vi "Test_ReadFast.vi"() -> (3 "Passed?":bool)   [LabVIEW 2017, in "WordManipulationTests.lvlib"]
uses:
  WordManipulationTests.lvlib
  SoftmotionClass/SoftmotionAxis/SoftmotionAxis.lvclass
  <vilib>/Motion/PropertyNodes/nimc.createStraightLineMoveInstance.axis.vi
  <vilib>/Motion/PropertyNodes/nimc.destroyInterfaceInstance.vi
  Utilities/WordManipulationLibrary.lvlib
  <resource>/objmgr/nimcai.rc
  Utilities/Bit Manipulation.lvlib
panel:
  out "appended array":dbl[](array[numeric])
  out "Velocity Feedback":dbl
  out "Position Feedback":dbl[](array[numeric])
  in  "Positions":dbl[](array[numeric])=[1000.0]
  in  "Velocity":dbl=1000.0
  in  "Acceleration":dbl=10000.0
  in  "Acceleration Jerk":dbl=1000.0
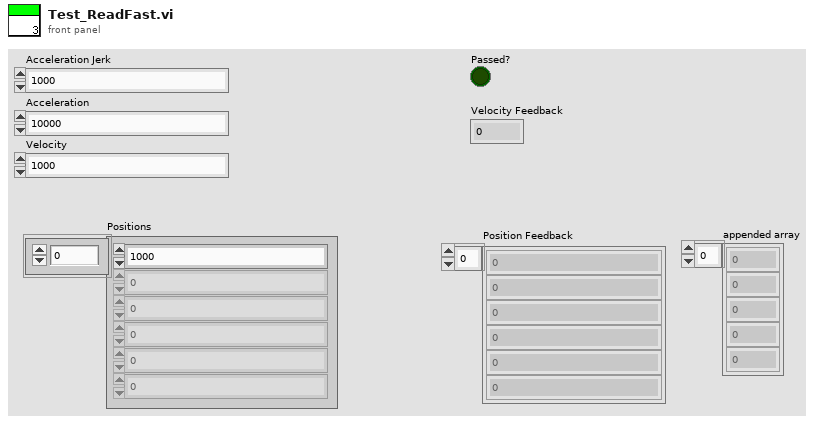
[diagram p1: front panel]
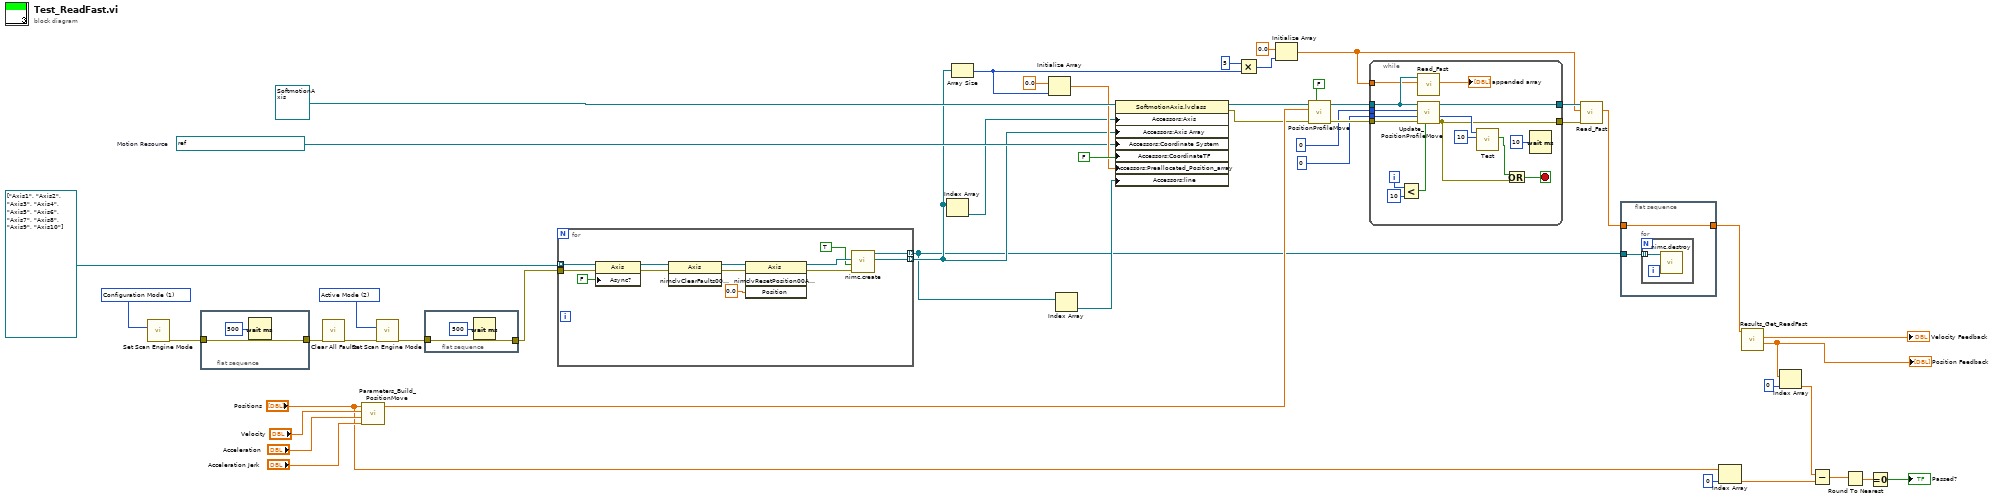
[diagram p0: block diagram]
diagram:
  w13 = 2 items=["Configuration Mode"=1, "Active Mode"=2] ("mode (Active Mode)")
  w15 = 1 items=["Configuration Mode"=1, "Active Mode"=2] ("mode (Active Mode)")
  w37 = refnum<k21> "nism://My Computer/Cord1"  # Motion Resource
  n1 = call <vilib>:"Set Scan Engine Mode.vi"("mode (Active Mode)"=w15) -> ("error out"=w12:errorcluster)  [unwired: 14 in]
  n2 = flat-sequence {
    tunnel: [w48] -> w11
    tunnel: w12 -> [w48]
    frame #0 {
      n3 = Wait (ms)(milliseconds to wait=u32 500) -> ()  [unwired: 1 out]
    }
  }
  n4 = call <vilib>:"Clear All Faults.vi"("error in (no error)"=w11) -> ("error out"=w10:errorcluster)  [unwired: 10 in]
  n5 = call "Parameters_Build_PositionMove.vi"("Acceleration Jerk"="Acceleration Jerk", "Acceleration"="Acceleration", "Velocity"="Velocity", "Positions"="Positions") -> ("Parameters"=w42:dbl[])  [unwired: 7 in]
  n6 = call <vilib>:"Set Scan Engine Mode.vi"("mode (Active Mode)"=w13, "error in (no error)"=w10) -> ("error out"=w9:errorcluster)  [unwired: 13 in]
  n7 = flat-sequence {
    tunnel: [w50] -> w14
    tunnel: w9 -> [w50]
    frame #0 {
      n8 = Wait (ms)(milliseconds to wait=u32 500) -> ()  [unwired: 1 out]
    }
  }
  n9 = for {
    tunnel: refnum<k21>[] ["Axis1", "Axis2", "Axis3", "Axis4", "Axis5", "Axis6", "Axis7", "Axis8", "Axis9", "Axis10"] ("Axis Array") -> [w63] mode=indexing
    tunnel: [w59] -> w21 mode=indexing
    tunnel: [w58] -> w20 mode=indexing
    tunnel: w14 -> [w57]
    n10 = property class="Axis"(reference=w63, error in=w57, "Async?"=FALSE) -> (reference out=w56:refnum<k21>, error out=w54:errorcluster)
    n11 = invoke class="Axis" method="nimclvClearFaults00A10001"(reference=w56, error in=w54) -> (reference out=w55:refnum<k21>, error out=w53:errorcluster)  [unwired: 1 in, 1 out]
    n12 = invoke class="Axis" method="nimclvResetPosition00A10001"(reference=w55, error in=w53, "Position"=0.0) -> (reference out=w61:refnum<k21>, error out=w52:errorcluster)  [unwired: 1 in, 2 out]
    n13 = call-poly <vilib>:"nimc.create.vi"("error in"=w52, "async?"=TRUE, "axis"=w61) -> ("axis out"=w59:refnum<k21>, "line"=w58:refnum<k20>)  [unwired: 6 in, 1 out]
  }
  n14 = Index Array(array=w21) -> (element=w22:refnum<k21>)  [unwired: 1 in]
  n15 = Array Size(array=w21) -> (size(s)=w30:i32)
  n16 = Initialize Array(0.0 ("element"), w30) -> (w44:dbl[])
  n17 = Index Array(array=w20) -> (element=w23:refnum<k20>)  [unwired: 1 in]
  n18 = property class="SoftmotionAxis.lvclass"(reference=refnum<class "SoftmotionAxis.lvclass"> refnum ("SoftmotionAxis in"), "Accessors:Axis"=w22, "Accessors:Axis Array"=w21, "Accessors:Coordinate System"=w37, "Accessors:CoordinateTF"=FALSE ("CoordinateTF"), "Accessors:Preallocated_Position_array"=w44, "Accessors:line"=w23) -> (reference out=w43:refnum<class "SoftmotionAxis.lvclass">, error out=w36:errorcluster)  [unwired: 1 in]
  n19 = Multiply(x=5, y=w30) -> (x*y=w28:i32)
  n20 = Initialize Array(0.0 ("element"), w28) -> (w8:dbl[])
  n21 = call-dynamic "PositionProfileMove.vi"("Relative?"=FALSE, "error in (no error)"=w36, "Array"=w42, "SoftmotionAxis in"=w43) -> ("error out"=w34:errorcluster, "SoftmotionAxis out"=w35:refnum<class "SoftmotionAxis.lvclass">)  [unwired: 6 in]
  n22 = while {
    tunnel: w35 -> [w71]
    tunnel: w34 -> [w80]
    tunnel: u16 0 ("ControlWord") -> [w79]
    tunnel: u16 0 ("StatusWord") -> [w78]
    tunnel: [w77] -> w31
    tunnel: [w72] -> w26
    tunnel: w8 -> [w69]
    i -> [w68]
    stop <- w73 stop-if-true
    n23 = Less?(x=w68, y=10) -> (x < y?=w66:bool)
    n24 = call-dynamic "Update_PositionProfileMove.vi"("Skip Update?"=w66, "error in (no error)"=w80, "StatusWord"=w78, "ControlWord"=w79, "SoftmotionAxis in"=w71) -> ("error out"=w72:errorcluster, "StatusWord Out"=w76:u16, "SoftmotionAxis out"=w77:refnum<class "SoftmotionAxis.lvclass">)  [unwired: 4 in]
    n25 = call-dynamic "Read_Fast.vi"("Results Array In"=w69, "SoftmotionAxis in"=w71) -> ("appended array"=→"appended array":dbl[])  [unwired: 7 in, 2 out]
    n26 = call "Test.vi"("Bit to test"=u8 10, "Data_In"=w76) -> ("bit value"=w74:bool)  [unwired: 8 in, 1 out]
    n27 = Or(x=w74, y=w72) -> (x .or. y?=w73:bool)
    n28 = Wait (ms)(milliseconds to wait=u32 10) -> ()  [unwired: 1 out]
  }
  n29 = call-dynamic "Read_Fast.vi"("error in (no error)"=w26, "Results Array In"=w8, "SoftmotionAxis in"=w31) -> ("appended array"=w1:dbl[])  [unwired: 6 in, 2 out]
  n30 = flat-sequence {
    tunnel: w20 -> [w82]
    tunnel: [w81] -> w2
    tunnel: w1 -> [w81]
    frame #0 {
      n31 = for {
        tunnel: w82 -> [w83] mode=indexing
        n32 = call-poly <vilib>:"nimc.destroy.vi"("motion handle"=w83) -> ()  [unwired: 10 in, 1 out]
      }
    }
  }
  n33 = Index Array(array="Positions", index=0) -> (element=w6:dbl)
  n34 = call "Results_Get_ReadFast.vi"("Results"=w2) -> ("Position"=w16:dbl[], "Velocity"=→"Velocity Feedback":dbl)  [unwired: 9 in]
  "Position Feedback" <- w16
  n35 = Index Array(array=w16, index=0) -> (element=w7:dbl)
  n36 = Subtract(x=w7, y=w6) -> (x-y=w5:dbl)
  n37 = Round To Nearest(number=w5) -> (nearest integer value=w4:dbl)
  n38 = Equal To 0?(x=w4) -> (x = 0?=→"Passed?":bool)
